vi "LDR midngt.vi"(0 "LINX Resource":T1, 1 "Trigger":u8, 3 "Trigger 2":u8, 5 "Error Out":errorcluster, 6 "Echo":u8, 10 "Echo 2":u8, 15 "IN2 Motor":u8, 16 "IN1 Motor":u8, 17 "Enable PWM Channel for  motor":u8, 18 "LDR Analog pin":u8) -> (4 "Waveform Chart u1\n 2":dbl(graph), 9 "Pulse Width (uS)":u32, 11 "Pulse Width (uS) 2":u32, 12 "U1 Distance(cm)":u32, 13 "U1 Distance(cm) 2":u32, 14 "LINX Resource 2":T1, 19 "Error Out 2":errorcluster)   [LabVIEW 2020]
uses:
  <vilib>/MakerHub/LINX/Private/Type Defs/LINX Ref.ctl
  <vilib>/MakerHub/LINX/Private/Type Defs/Platform.ctl
  <vilib>/MakerHub/LINX/Private/Type Defs/Interface.ctl
  <vilib>/MakerHub/LINX/Private/Device/Type Defs/LINX Device Config.ctl
  <vilib>/MakerHub/LINX/Private/Device/Type Defs/TCP Config.ctl
  <vilib>/MakerHub/LINX/Private/Device/Type Defs/Channels.ctl
  <vilib>/MakerHub/LINX/Private/Device/Type Defs/Stimulus Pulse.ctl
  <vilib>/MakerHub/LINX/Public/Peripherals/Analog/Analog Read 1 Chan.vi
  <vilib>/MakerHub/LINX/Public/Peripherals/Digital/Digital Write 1 Chan.vi
  <vilib>/MakerHub/LINX/Public/Peripherals/PWM/PWM Set Duty Cycle 1 Chan.vi
  <vilib>/MakerHub/LINX/Public/Peripherals/Analog/Analog Read N Chans.vi
  <vilib>/MakerHub/LINX/Public/Peripherals/Digital/Digital Write N Chans.vi
  <vilib>/MakerHub/LINX/Private/Local IO/LinxAnalogRead.vi
  <vilib>/MakerHub/LINX/Public/Utilities/Check Channel.vi
  <vilib>/MakerHub/LINX/Private/Local IO/LinxDigitalWrite.vi
  <vilib>/MakerHub/LINX/Private/Utilties/Generate Error.vi
  <vilib>/MakerHub/LINX/Public/Peripherals/PWM/PWM Set Duty Cycle N Chans.vi
  <vilib>/MakerHub/LINX/Private/Device/Device.lvlib
  <vilib>/MakerHub/LINX/LMH-LINX.lvlib
panel:
  out "Light Intensity":dbl
  out "voltage across ldr":dbl
  in  "Knob":dbl(knob) scale=0.0..1.0
  out "Waveform Chart u1":dbl(graph)
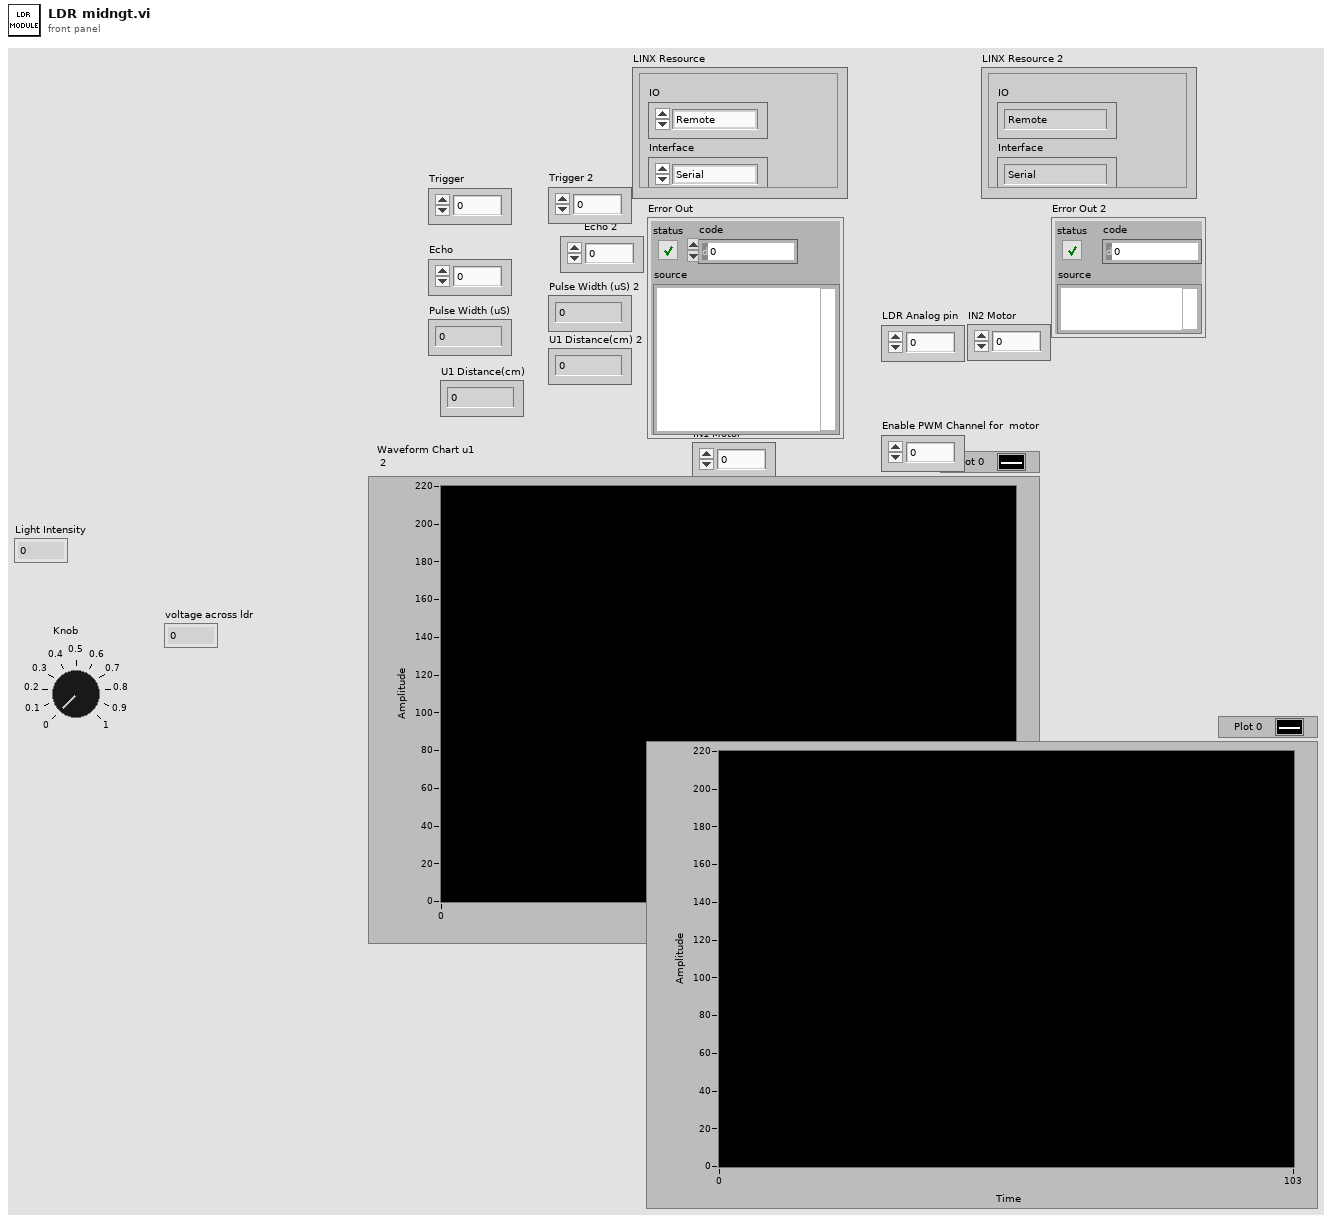
[diagram p1: front panel]
types:
  T1 = typedef "LMH-LINX.lvlib/LINX Ref.ctl" = cluster{"IO":T2, "Interface":T3, "LINX Device Config":T4}
  T2 = typedef "LMH-LINX.lvlib/Platform.ctl" = enum16{"Remote", "Local"}
  T3 = typedef "LMH-LINX.lvlib/Interface.ctl" = enum16{"Serial", "TCP"}
  T4 = typedef "LMH-LINX.lvlib/Device.lvlib/LINX Device Config.ctl" = cluster{"Interface":T3, "COM Port":refnum<visa-resource-name>, "TCP Configuration":T5, "Device Family":u8, "Device ID":u8, "Device Name":string, "TCP Ref":refnum<k5>, "Channels":T6}
  T5 = typedef "LMH-LINX.lvlib/Device.lvlib/TCP Config.ctl" = cluster{"IP Address":string, "Port":u16}
  T6 = typedef "LMH-LINX.lvlib/Channels.ctl" = cluster{"DI":u8[], "DO":u8[], "AI":u8[], "AO":u8[], "PWM":u8[], "QE":u8[], "UART":u8[], "I2C 2":u8[], "SPI":u8[], "CAN":u8[], "Servo":u8[], "AI Ref (V)":dbl, "AI Resolution (Bits)":u8, "AO Ref (V)":dbl, "AO Resolution (Bits)":u8}
  T7 = typedef "LMH-LINX.lvlib/Device.lvlib/Stimulus Pulse.ctl" = enum16{"None", "Active Low", "Active High"}
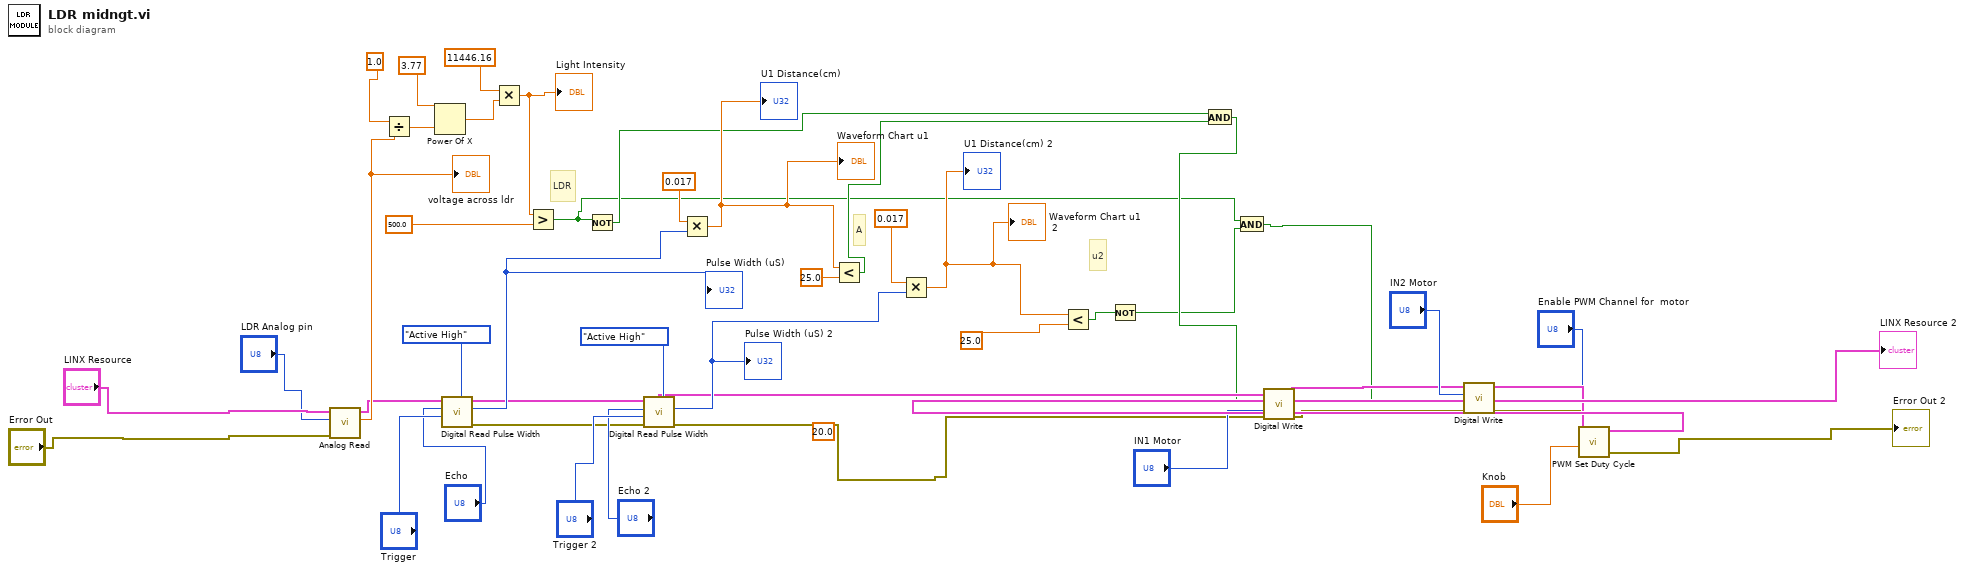
[diagram p0: block diagram]
diagram:
  (unwired) 20.0 ("Time Target (s)")
  # "u2"
  # "A"
  # "LDR"
  n1 = call-poly <vilib>:"Analog Read.vi"("Error In"="Error Out", "Analog Channel"="LDR Analog pin", "LINX Resource"="LINX Resource") -> ("Voltage"=w38:dbl, "LINX Resource"=w27:T1)  [unwired: 5 in, 2 out]
  "voltage across ldr" <- w38
  n2 = Divide(x=1.0, y=w38) -> (x/y=w42:dbl)
  n3 = Power Of X(1:w42, 2:3.77 ("y")) -> (0:w40:dbl)
  n4 = call <vilib>:"Digital Read Pulse Width.vi"("Stimulus Pulse (Active High)"=Stimulus_Pulse."Active High", "DO Channel"="Trigger", "DI Channel"="Echo", "LINX Resource"=w27) -> ("Error Out"=w12:errorcluster, "Pulse Width (uS)"=w32:u32, "LINX Resource"=w13:T1)  [unwired: 5 in]
  "Pulse Width (uS)" <- w32
  n5 = Multiply(x=11446.16, y=w40) -> (x*y=w26:dbl)
  "Light Intensity" <- w26
  n6 = Greater?(x=w26, y=500.0) -> (0:w3:bool)
  n7 = Not(x=w3) -> (.not. x?=w8:bool)
  n8 = call <vilib>:"Digital Read Pulse Width.vi"("Stimulus Pulse (Active High)"=Stimulus_Pulse."Active High", "Error In"=w12, "DO Channel"="Trigger 2", "DI Channel"="Echo 2", "LINX Resource"=w13) -> ("Error Out"=w1:errorcluster, "Pulse Width (uS)"=w15:u32, "LINX Resource"=w11:T1)  [unwired: 4 in]
  "Pulse Width (uS) 2" <- w15
  n9 = Multiply(x=0.017, y=w32) -> (x*y=w31:dbl)
  "U1 Distance(cm)" <- w31
  "Waveform Chart u1" <- w31
  n10 = Less?(x=w31, y=25.0) -> (x < y?=w7:bool)
  n11 = Multiply(x=0.017, y=w15) -> (x*y=w17:dbl)
  "U1 Distance(cm) 2" <- w17
  "Waveform Chart u1\n 2" <- w17
  n12 = Less?(x=w17, y=25.0) -> (x < y?=w4:bool)
  n13 = Not(x=w4) -> (.not. x?=w2:bool)
  n14 = And(x=w8, y=w7) -> (x .and. y?=w6:bool)
  n15 = And(x=w3, y=w2) -> (x .and. y?=w5:bool)
  n16 = call-poly <vilib>:"Digital Write.vi"("Error In"=w1, "Output Value"=w6, "DO Channel"="IN1 Motor", "LINX Resource"=w11) -> ("Error Out"=w9:errorcluster, "LINX Resource"=w10:T1)  [unwired: 6 in]
  n17 = call-poly <vilib>:"Digital Write.vi"("Error In"=w9, "Output Value"=w5, "DO Channel"="IN2 Motor", "LINX Resource"=w10) -> ("Error Out"=w36:errorcluster, "LINX Resource"=w37:T1)  [unwired: 6 in]
  n18 = call-poly <vilib>:"PWM Set Duty Cycle.vi"("Error In"=w36, "Duty Cycle (0-1)"="Knob", "PWM Channel"="Enable PWM Channel for  motor", "LINX Resource"=w37) -> ("Error Out"=→"Error Out 2":errorcluster, "LINX Resource"=→"LINX Resource 2":T1)  [unwired: 6 in]
